vi "Offline_Analysis__SWLDA_분석기.vi"(0 "LDA_matrix":path=path "C:/Emotion_Research/ABM_Analysis/ABM_Analysis_Data_150304/OhJinHyuk_ABM_150305/ABM_150305_Training_Test(LDA)/2014-03-05/SWLDA/LDA_Matrix_Value_SWLDA_pe005pr01.txt" caption="LDA_matrix.txt", 5 "Weight":path=path "C:/Emotion_Research/ABM_Analysis/ABM_Analysis_Data_150304/OhJinHyuk_ABM_150305/ABM_150305_Training_Test(LDA)/2014-03-05/SWLDA/Weight_Vector_SWLDA_pe005pr01.txt" caption="weight.txt", 7 "Target_order.txt":path=path "C:/Emotion_Research/ABM_Analysis/ABM_Analysis_Data_150304/OhJinHyuk_ABM_150305/ABM_150305_Online(Step2)/2014-03-05/Target_order.txt", 9 "mius_flash_order":path=path "C:/Emotion_Research/ABM_Analysis/ABM_Analysis_Data_150304/OhJinHyuk_ABM_150305/ABM_150305_Online(Step2)/2014-03-05/mius_flash_order.txt", 11 "Brain":path=path "C:/Emotion_Research/ABM_Analysis/ABM_Analysis_Data_150304/OhJinHyuk_ABM_150305/ABM_150305_Online(Step2)/2014-03-05/Brain.txt", 12 "피험자이름":string="오진혁_SWLDA_LDA_pe005pr01", 13 "Save_path":string="Emotion_Research\\Result") -> ()   [LabVIEW 2014]
uses:
  <vilib>/Utility/file.llb/Read From Spreadsheet File (DBL).vi
  <vilib>/Analysis/Matrix/Numeric/Conversions/Array To Matrix - RA2.vi
  <vilib>/Analysis/Matrix/Numeric/Conversions/Array To Matrix - RA.vi
  <vilib>/Utility/file.llb/Read From Spreadsheet File (I64).vi
  <vilib>/Utility/file.llb/Write To Spreadsheet File (DBL).vi
  <vilib>/Utility/file.llb/Write To Spreadsheet File (I64).vi
  <vilib>/Utility/file.llb/Write To Spreadsheet File (string).vi
  <vilib>/Analysis/Matrix/NI_Matrix.lvlib
panel:
  out "ACC":i16
  in  "Channel selection":bool[](array[boolean])=[TRUE, TRUE, TRUE, TRUE, TRUE, TRUE, TRUE, TRUE, TRUE, TRUE, TRUE]
  out "Target_order":i64[](array[numeric])
  out "Selected_Target":i32[](array[numeric])
  out "Accuracy":i16[](array[numeric])
  in  "사용할 Parameter 갯수":i32=44
  out "error out":errorcluster={"status"=TRUE, "code"=10, "source"="Create Folder in Offline_Analysis__SWLDA_분석기.vi->분석기_v2.vi<APPEND>\nC:\\Emotion_Research\\ABM_Analysis\\ABM_Analysis_Data_150304\\OhJinHyuk_ABM_150305\\Test_Result\\오진혁_SWLDA_LDA_pe005pr01"}
  in  "Random_num":i32=6
  in  "Flash_Repeat":i32=20
  in  "Frame_Length":i32=10
  in  "Sampling_Rate":dbl=250.0
  in  "ERP_Parameters_of_NonTarget":path caption="ERP_Parameters_of_NonTarget.txt"
  in  "ERP_Parameters_of_Target":path caption="ERP_Parameters_of_Target.txt"
  # "ERP_Parameter안씀. LDA바로 집어넣으면 됨"
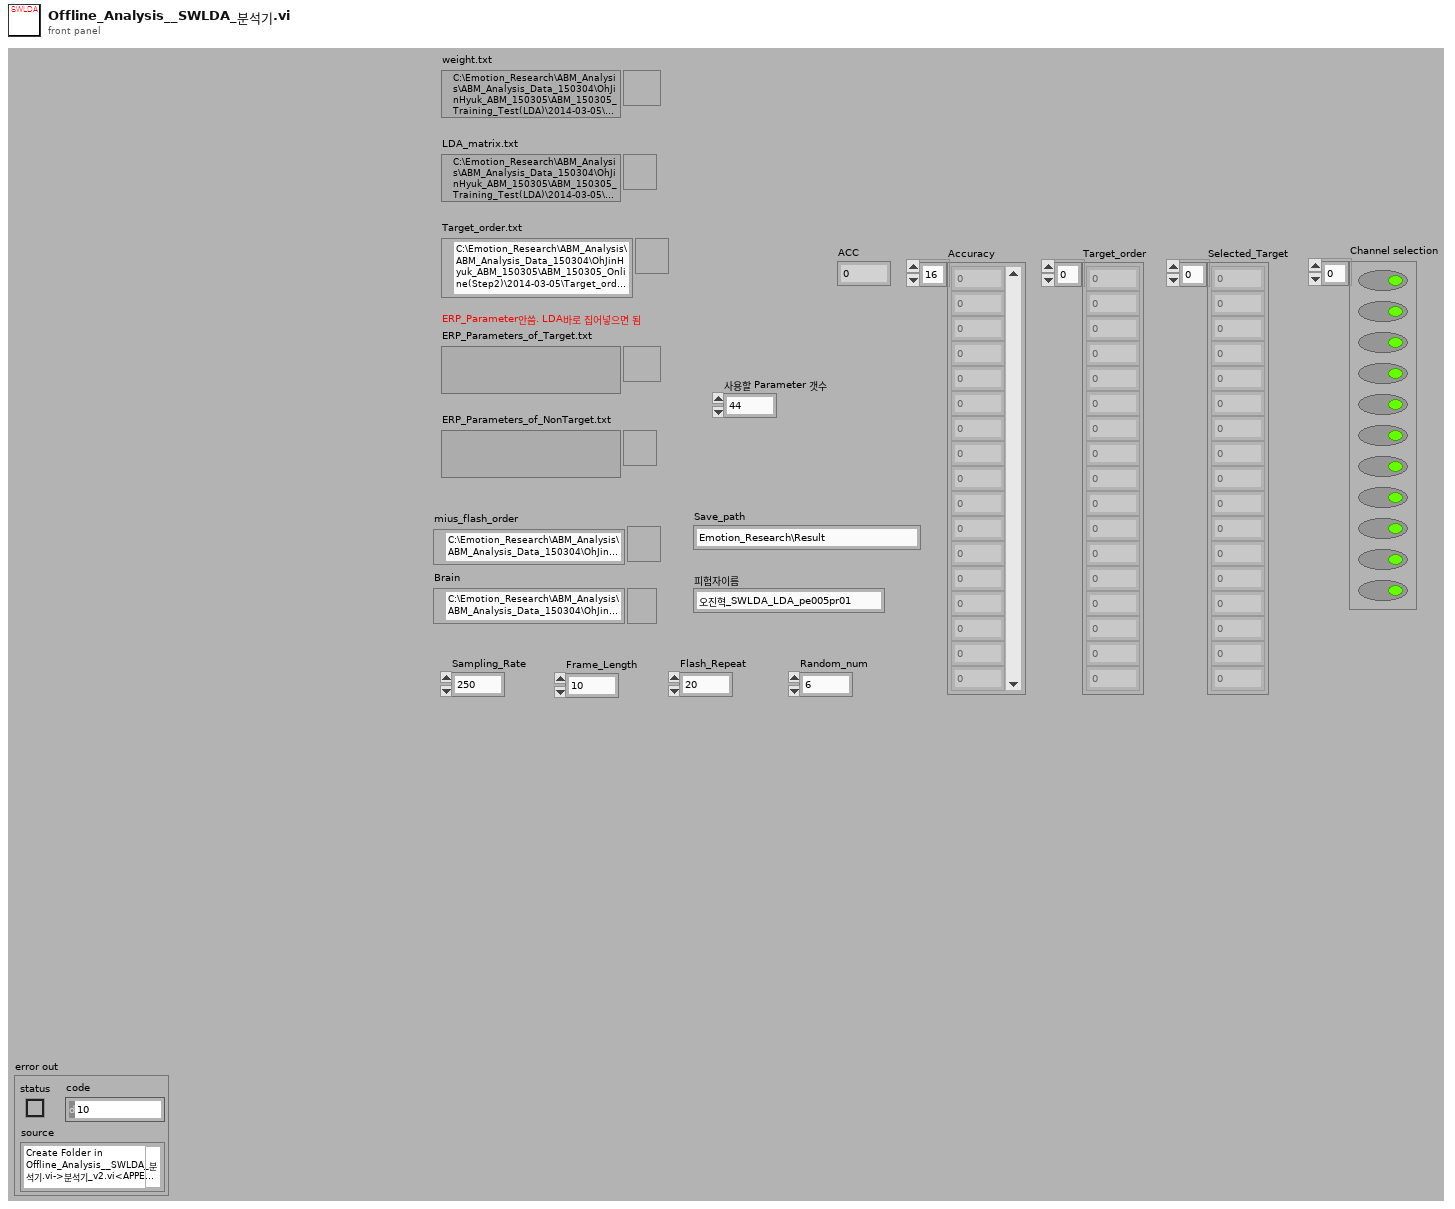
[diagram p1: front panel]
types:
  T1 = typedef "NI_Matrix.lvlib/RealMatrix.ctl" = dbl[][]
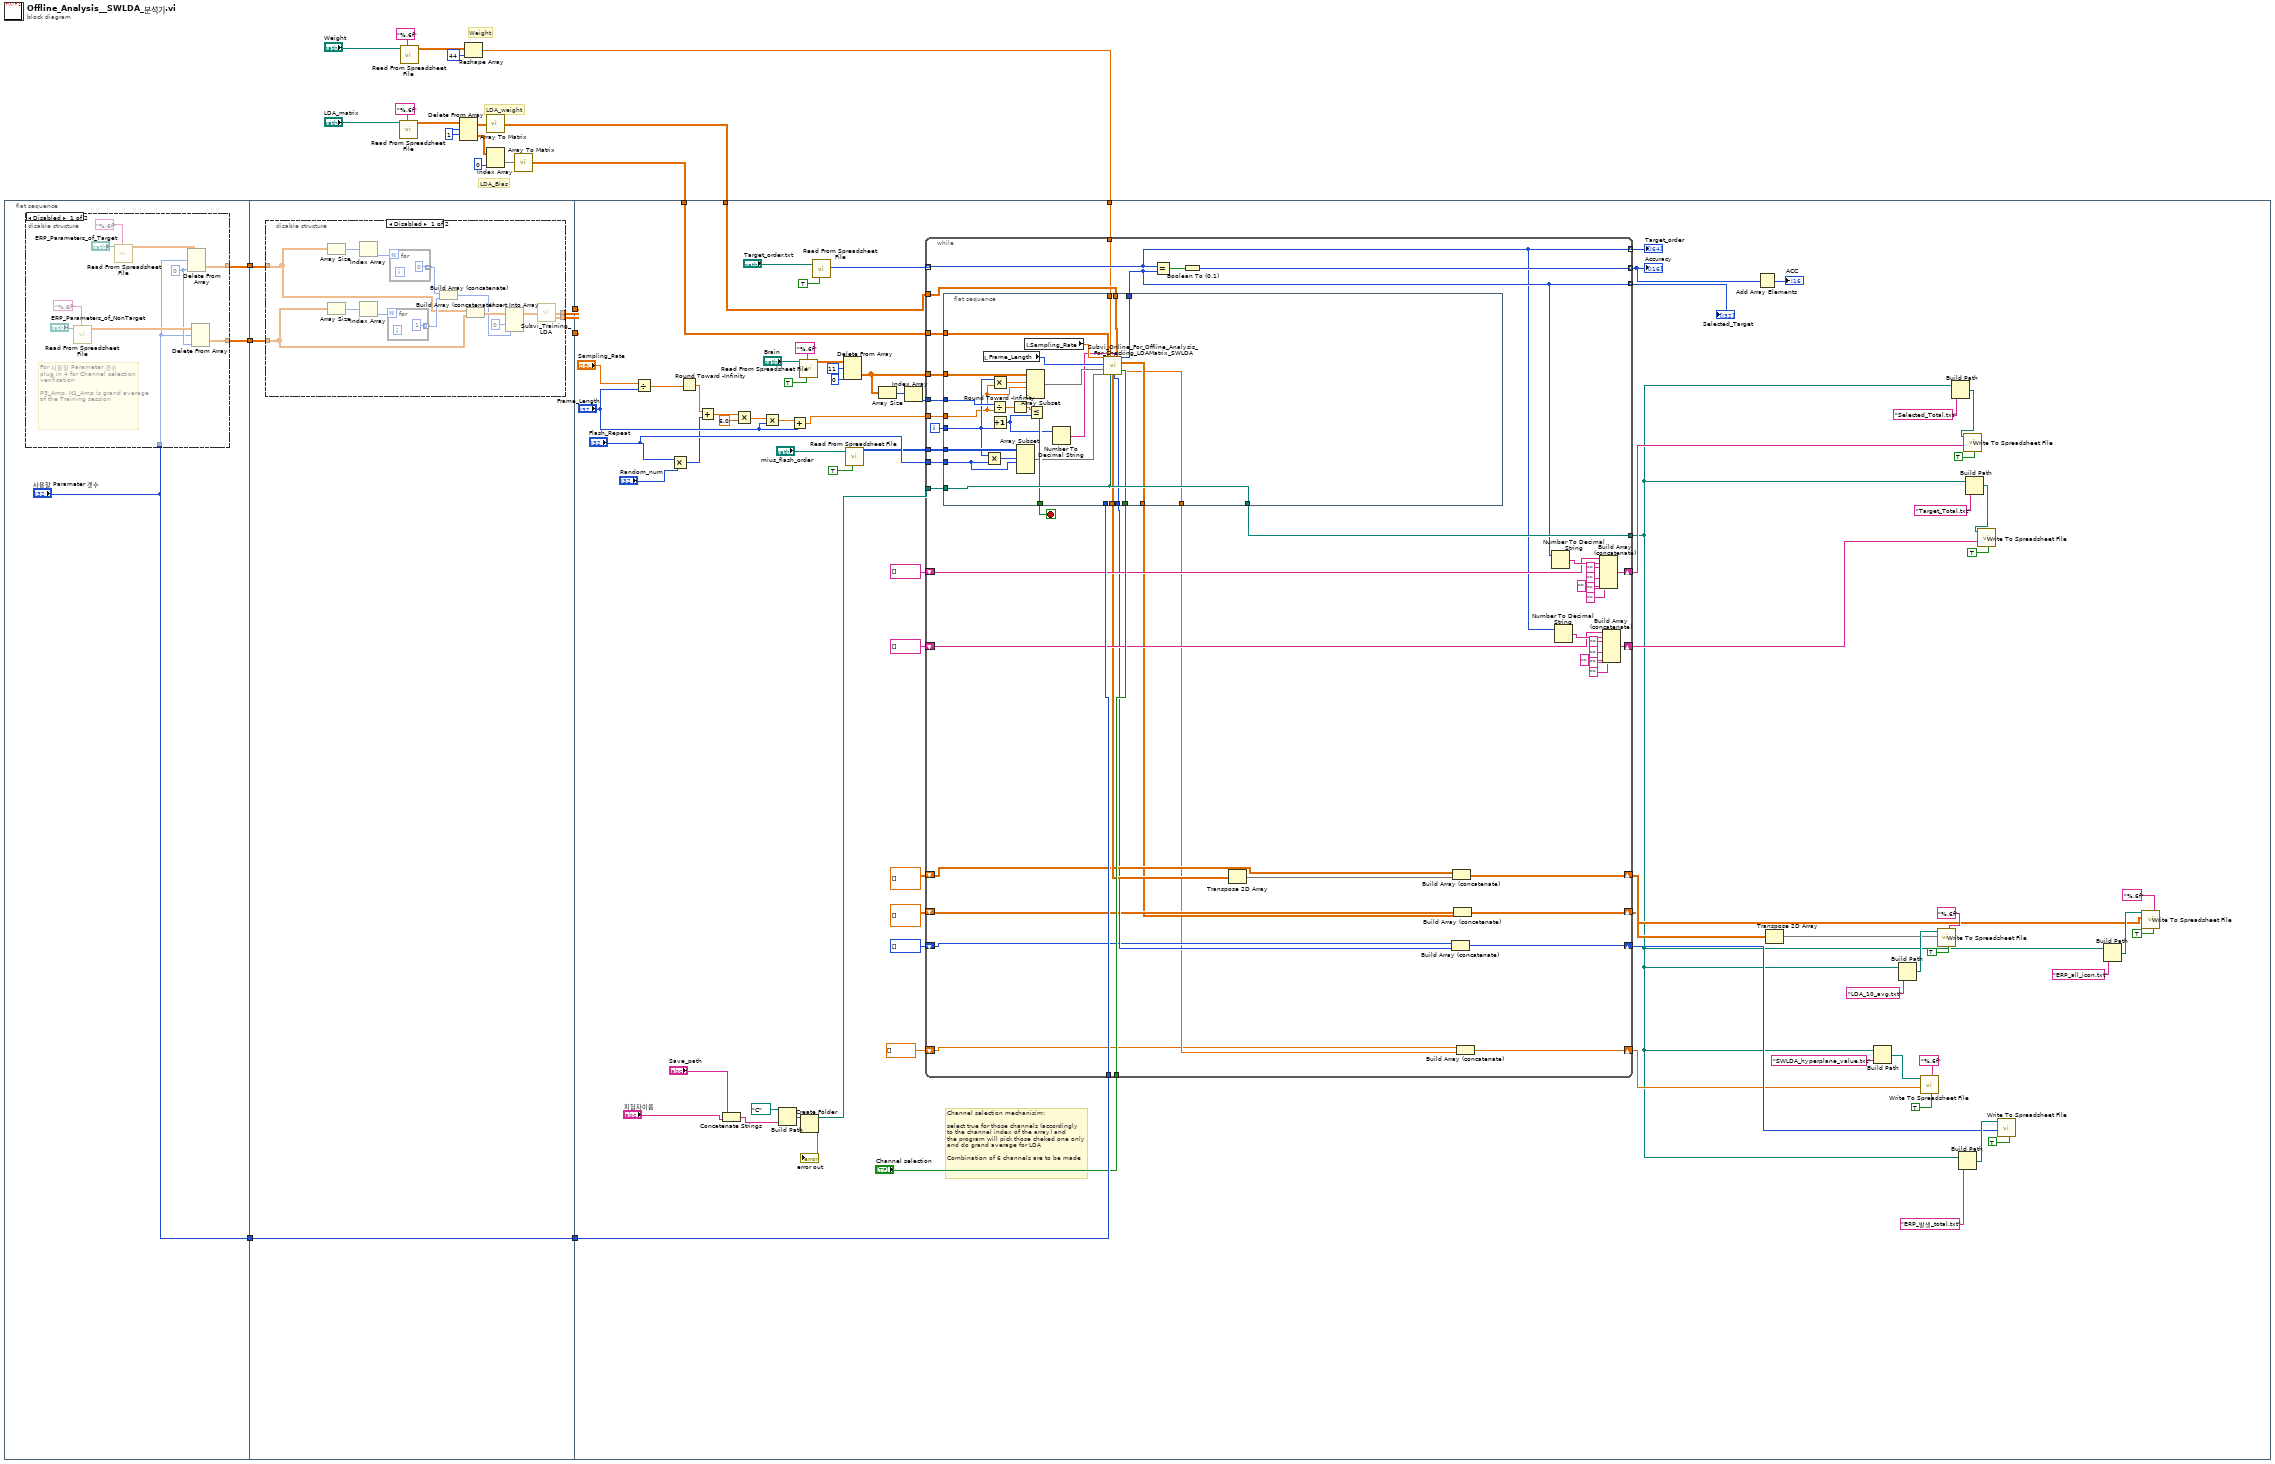
[diagram p0: block diagram]
diagram:
  w10 = 1 ("인덱스 (행)")
  # "LDA_Bias"
  # "LDA_weight"
  # "Weight"
  n1 = flat-sequence {
    tunnel: [w24] -> w21
    tunnel: [w23] -> w20
    tunnel: ["사용할 Parameter 갯수"] -> w17
    tunnel: w21 -> [w39]
    tunnel: w20 -> [w38]
    tunnel: [w37] -> w19
    tunnel: [w36] -> w18
    tunnel: w17 -> [w35]
    tunnel: [w35] -> w16
    tunnel: w19 -> [_]
    tunnel: w18 -> [_]
    tunnel: w16 -> [w105]
    tunnel: w7 -> [w74]
    tunnel: w6 -> [w73]
    tunnel: w2 -> [w72]
    frame #0 {
      n2 = disable-structure shown="Disabled" {
        disable-tunnel: [w27 _] -> w24
        disable-tunnel: [w26 _] -> w23
        disable-tunnel: "사용할 Parameter 갯수" -> [w25 _]
        frame Disabled {
          w28 = 0 ("비활성화된 인덱스 (열)")
          # "For 사용할 Parameter 갯수\nplug in 4 for Channel selection\nverification\n\nP3_Amp, N1_Amp is grand average of the Training session"
          n3 = call-poly <vilib>:"Read From Spreadsheet File.vi"("format (%.3f)"="%.6f", "file path (dialog if empty)"="ERP_Parameters_of_NonTarget") -> ("all rows"=w29:dbl[][])  [unwired: 5 in, 4 out]
          n4 = call-poly <vilib>:"Read From Spreadsheet File.vi"("format (%.3f)"="%.6f", "file path (dialog if empty)"="ERP_Parameters_of_Target") -> ("all rows"=w30:dbl[][])  [unwired: 5 in, 4 out]
          n5 = Delete From Array(array=w30, length=w25, index (col)=w28) -> (deleted portion=w27:dbl[][])  [unwired: 1 in, 1 out]
          n6 = Delete From Array(array=w29, length=w25, index (col)=w28) -> (deleted portion=w26:dbl[][])  [unwired: 1 in, 1 out]
        }
        frame Enabled {
        }
      }
    }
    frame #1 {
      n7 = disable-structure shown="Disabled" {
        disable-tunnel: w39 -> [w44 _]
        disable-tunnel: w38 -> [w43 _]
        disable-tunnel: [w42 _] -> w37
        disable-tunnel: [w41 _] -> w36
        frame Disabled {
          n8 = Array Size(array=w44) -> (size(s)=w48:i32[])
          n9 = Array Size(array=w43) -> (size(s)=w49:i32[])
          n10 = Index Array(array=w48) -> (element=w50:i32)  [unwired: 1 in]
          n11 = Index Array(array=w49) -> (element=w51:i32)  [unwired: 1 in]
          n12 = for {
            N: w51 -> [_]
            tunnel: [1] -> w53 mode=indexing
          }
          n13 = for {
            N: w50 -> [_]
            tunnel: [0] -> w52 mode=indexing
          }
          n14 = Build Array (concatenate)(w52, w53) -> (w45:i32[])
          n15 = Build Array (concatenate)(w44, w43) -> (w46:dbl[][])
          n16 = Insert Into Array(array=w46, index (col)=0 ("비활성화된 인덱스 (열)"), new element=w45) -> (w40:dbl[][])  [unwired: 1 in]
          n17 = call "Subvi_Training_LDA.vi"("Input_Data"=w40) -> ("A * B 2"=w42:T1, "A * B"=w41:T1)
        }
        frame Enabled {
        }
      }
    }
    frame #2 {
      # "Channel selection mechanisim:\n\nselect true for those channels (accordingly\nto the channel index of the array) and \nthe program will pick those cheked one only\nand do grand average for LDA\n\nCombination of 6 channels are to be made"
      n18 = Divide(x="Sampling_Rate", y="Frame_Length") -> (x/y=w117:dbl)
      n19 = Multiply(x="Flash_Repeat", y="Random_num") -> (x*y=w120:i32)
      n20 = Round Toward -Infinity(1:w117) -> (0:w119:dbl)
      n21 = Add(x=w119, y=w120) -> (x+y=w122:dbl)
      n22 = Concatenate Strings("Save_path", "피험자이름") -> (w58:string)
      n23 = Multiply(x=w122, y=6.0) -> (x*y=w124:dbl)
      n24 = Multiply(x=w124, y="Frame_Length") -> (x*y=w126:dbl)
      n25 = Build Path(base path=path "C:/" ("path"), name or relative path=w58) -> (appended path=w129:path)
      n26 = Add(x=w126, y="Frame_Length") -> (x+y=w127:dbl)
      n27 = call-poly <vilib>:"Read From Spreadsheet File.vi"("transpose (no:F)"=TRUE, "format (%.3f)"="%.6f", "file path (dialog if empty)"="Brain") -> ("all rows"=w110:dbl[][])  [unwired: 4 in, 4 out]
      n28 = Create Folder(path (use dialog)=w129) -> (created path=w131:path, error out=→"error out":errorcluster)  [unwired: 2 in, 1 out]
      n29 = call-poly <vilib>:"Read From Spreadsheet File.vi"("transpose (no:F)"=TRUE, "file path (dialog if empty)"="Target_order.txt") -> ("first row"=w103:i64[])  [unwired: 5 in, 4 out]
      n30 = Delete From Array(array=w110, length=11 ("길이"), index (col)=0 ("비활성화된 인덱스 (열)")) -> (deleted portion=w113:dbl[][])  [unwired: 1 in, 1 out]
      n31 = call-poly <vilib>:"Read From Spreadsheet File.vi"("transpose (no:F)"=TRUE, "file path (dialog if empty)"="mius_flash_order") -> ("all rows"=w112:i64[][])  [unwired: 5 in, 4 out]
      n32 = Array Size(array=w113) -> (size(s)=w114:i32[])
      n33 = Index Array(array=w114) -> (element=w115:i32)  [unwired: 1 in]
      n34 = while {
        tunnel: w73 -> [w180]
        tunnel: w74 -> [w179]
        tunnel: w113 -> [w177]
        tunnel: w112 -> [w176]
        tunnel: w115 -> [w178]
        tunnel: w127 -> [w174]
        tunnel: "Flash_Repeat" -> [w175]
        tunnel: w131 -> [w173]
        tunnel: w105 -> [w172]
        tunnel: w103 -> [w150] mode=indexing
        tunnel: [w170] -> w94 mode=indexing
        tunnel: [w150] -> w100 mode=indexing
        tunnel: [w151] -> w101 mode=indexing
        tunnel: "Channel selection" -> [w167]
        tunnel: [w166] -> w59
        shift-right: [w153] -> w88
        shift-left: string[] [] -> [w152]
        shift-right: [w149] -> w87
        shift-left: string[] [] -> [w148]
        shift-right: [w145] -> w80
        shift-left: dbl[][] [] -> [w144]
        shift-right: [w142] -> w75
        shift-left: i16[] [] -> [w141]
        tunnel: w72 -> [w140]
        shift-right: [w139] -> w66
        shift-left: dbl[][] [] -> [w138]
        shift-right: [w135] -> w60
        shift-left: dbl[] [] -> [w134]
        i -> [w169]
        stop <- w168 stop-if-true
        n35 = flat-sequence {
          tunnel: [w207] -> w166
          tunnel: [w182] -> w137
          tunnel: w140 -> [w183]
          tunnel: [w184] -> w143
          tunnel: [w185] -> w146
          tunnel: w167 -> [w187]
          tunnel: [w188] -> w151
          tunnel: w172 -> [_]
          tunnel: w173 -> [w207]
          tunnel: w174 -> [w194]
          tunnel: w169 -> [w195]
          tunnel: w175 -> [w197]
          tunnel: w176 -> [w199]
          tunnel: w177 -> [w202]
          tunnel: [w203] -> w168
          tunnel: w178 -> [w204]
          tunnel: w179 -> [w205]
          tunnel: w180 -> [w206]
          tunnel: [w181] -> w136
          frame #0 {
            n36 = local read "Frame_Length"() -> (w190:i32)
            n37 = Multiply(x=w195, y=w197) -> (x*y=w198:i32)
            n38 = Divide(x=w204, y=w194) -> (x/y=w193:dbl)
            n39 = Multiply(x=w195, y=w194) -> (x*y=w201:dbl)
            n40 = Increment(x=w195) -> (x+1=w189:i32)
            n41 = Round Toward -Infinity(1:w193) -> (0:w192:dbl)
            n42 = Array Subset(array=w199, index (row)=w198, length (row)=w197) -> (w196:i64[][])  [unwired: 2 in]
            n43 = local read "Sampling_Rate"() -> (w191:dbl)
            n44 = Array Subset(array=w202, index (row)=w201, length (row)=w194) -> (w200:dbl[][])  [unwired: 2 in]
            n45 = Less Or Equal?(x=w192, y=w189) -> (x <= y?=w203:bool)
            n46 = Number To Decimal String(number=w189) -> (decimal integer string=w186:string)  [unwired: 1 in]
            n47 = call "Subvi_Online_For_Offline_Analysis_For_Checking_LDAMatrix_SWLDA.vi"("rate"=w191, "samples per channel"=w190, "Brain_data_source"=w200, "Target_Flash_Order"=w196, "Value"=w206, "Weight"=w183, "Path"=w207, "Number"=w186, "Matrix"=w205, "Channel selection"=w187) -> ("LDA_Parameter"=w185:dbl[][], "EPR_발생_total"=w184:i16[], "output-0~8"=w188:i32, "ERP_Parameters"=w182:dbl[][], "SWLDA"=w181:dbl[])  [unwired: 13 in]
          }
        }
        n48 = Equal?(x=w150, y=w151) -> (x = y?=w171:bool)
        n49 = Boolean To (0,1)(Boolean=w171) -> (0, 1=w170:i16)
        n50 = Transpose 2D Array(2D array=w146) -> (transposed array=w147:dbl[][])
        n51 = Build Array (concatenate)(w141, w143) -> (w142:i16[])
        n52 = Build Array (concatenate)(w144, w147) -> (w145:dbl[][])
        n53 = Build Array (concatenate)(w138, w137) -> (w139:dbl[][])
        n54 = Build Array (concatenate)(w134, w136) -> (w135:dbl[])
        n55 = Number To Decimal String(number=w151) -> (decimal integer string=w159:string)  [unwired: 1 in]
        n56 = Number To Decimal String(number=w150) -> (decimal integer string=w165:string)  [unwired: 1 in]
        n57 = Build Array (concatenate)(w152, w159, "" ("element"), "" ("element"), "" ("element"), "" ("element"), "" ("element")) -> (w153:string[])
        n58 = Build Array (concatenate)(w148, w165, "" ("element"), "" ("element"), "" ("element"), "" ("element"), "" ("element")) -> (w149:string[])
      }
      "Accuracy" <- w94
      "Selected_Target" <- w101
      "Target_order" <- w100
      n59 = Add Array Elements(numeric array=w94) -> (sum=→"ACC":i16)
      n60 = Transpose 2D Array(2D array=w80) -> (transposed array=w81:dbl[][])
      n61 = Build Path(base path=w59, name or relative path="SWLDA_hyperplane_value.txt") -> (appended path=w61:path)
      n62 = Build Path(base path=w59, name or relative path="LDA_10_avg.txt") -> (appended path=w83:path)
      n63 = call-poly <vilib>:"Write To Spreadsheet File.vi"("transpose? (no:F)"=TRUE, "format (%.3f)"="%.6f", "1D data"=w60, "file path (dialog if empty)"=w61) -> ()  [unwired: 4 in, 1 out]
      n64 = call-poly <vilib>:"Write To Spreadsheet File.vi"("transpose? (no:F)"=TRUE, "format (%.3f)"="%.6f", "2D data"=w81, "file path (dialog if empty)"=w83) -> ()  [unwired: 4 in, 1 out]
      n65 = Build Path(base path=w59, name or relative path="Selected_Total.txt") -> (appended path=w90:path)
      n66 = Build Path(base path=w59, name or relative path="ERP_발생_total.txt") -> (appended path=w77:path)
      n67 = call-poly <vilib>:"Write To Spreadsheet File.vi"("transpose? (no:F)"=TRUE, "1D data"=w88, "file path (dialog if empty)"=w90) -> ()  [unwired: 5 in, 1 out]
      n68 = Build Path(base path=w59, name or relative path="Target_Total.txt") -> (appended path=w96:path)
      n69 = call-poly <vilib>:"Write To Spreadsheet File.vi"("transpose? (no:F)"=TRUE, "1D data"=w87, "file path (dialog if empty)"=w96) -> ()  [unwired: 5 in, 1 out]
      n70 = call-poly <vilib>:"Write To Spreadsheet File.vi"("transpose? (no:F)"=TRUE, "1D data"=w75, "file path (dialog if empty)"=w77) -> ()  [unwired: 5 in, 1 out]
      n71 = Build Path(base path=w59, name or relative path="ERP_all_icon.txt") -> (appended path=w69:path)
      n72 = call-poly <vilib>:"Write To Spreadsheet File.vi"("transpose? (no:F)"=TRUE, "format (%.3f)"="%.6f", "2D data"=w66, "file path (dialog if empty)"=w69) -> ()  [unwired: 4 in, 1 out]
    }
  }
  n73 = call-poly <vilib>:"Read From Spreadsheet File.vi"("format (%.3f)"="%.6f", "file path (dialog if empty)"="LDA_matrix") -> ("all rows"=w8:dbl[][])  [unwired: 5 in, 4 out]
  n74 = call-poly <vilib>:"Read From Spreadsheet File.vi"("format (%.3f)"="%.6f", "file path (dialog if empty)"="Weight") -> ("all rows"=w3:dbl[][])  [unwired: 5 in, 4 out]
  n75 = Delete From Array(array=w8, length=w10, index (row)=w10) -> (deleted portion=w13:dbl[][], array with subset deleted=w12:dbl[][])  [unwired: 1 in]
  n76 = Reshape Array(w3, 44 ("dimension size")) -> (w2:dbl[])
  n77 = call-poly <vilib>:"Array To Matrix.vi"("Real 2D Array"=w12) -> ("Real Matrix"=w7:T1)
  n78 = Index Array(array=w13, index (col)=0 ("인덱스")) -> (element=w11:dbl[])  [unwired: 1 in]
  n79 = call-poly <vilib>:"Array To Matrix.vi"("Real 1D Array"=w11) -> ("Real Matrix (Column Vector)"=w6:T1)
